vi "RVHR - UI Values.vi"(4 "Default Reporting Settings":T1, 5 "Units":u8, 6 "Initialise?":bool, 7 "Command":enum16{"Set", "Get"}(ring), 8 "error in (no error)":errorcluster, 10 "Reporting IN":T1, 11 "UI Refs":T2) -> (0 "error out":errorcluster, 2 "Reporting Out":T1)   [LabVIEW 2024]
uses:
  Controls/RVHR - Reporting Settings.ctl
  Controls/RVHR - Setting refs.ctl
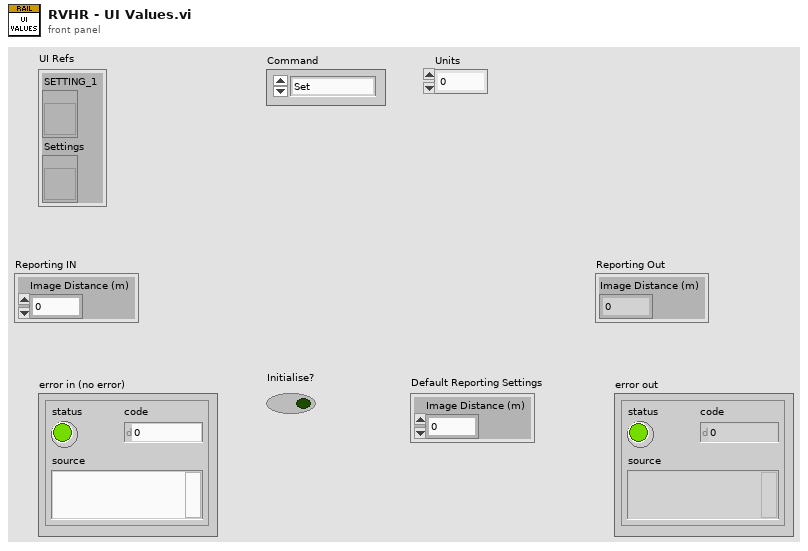
[diagram p1: front panel]
types:
  T1 = typedef "RVHR - Reporting Settings.ctl" = cluster{"Image Distance (m)":dbl}
  T2 = typedef "RVHR - Setting refs.ctl" = cluster{"SETTING_1":refnum<vi>, "Settings":refnum<vi>}
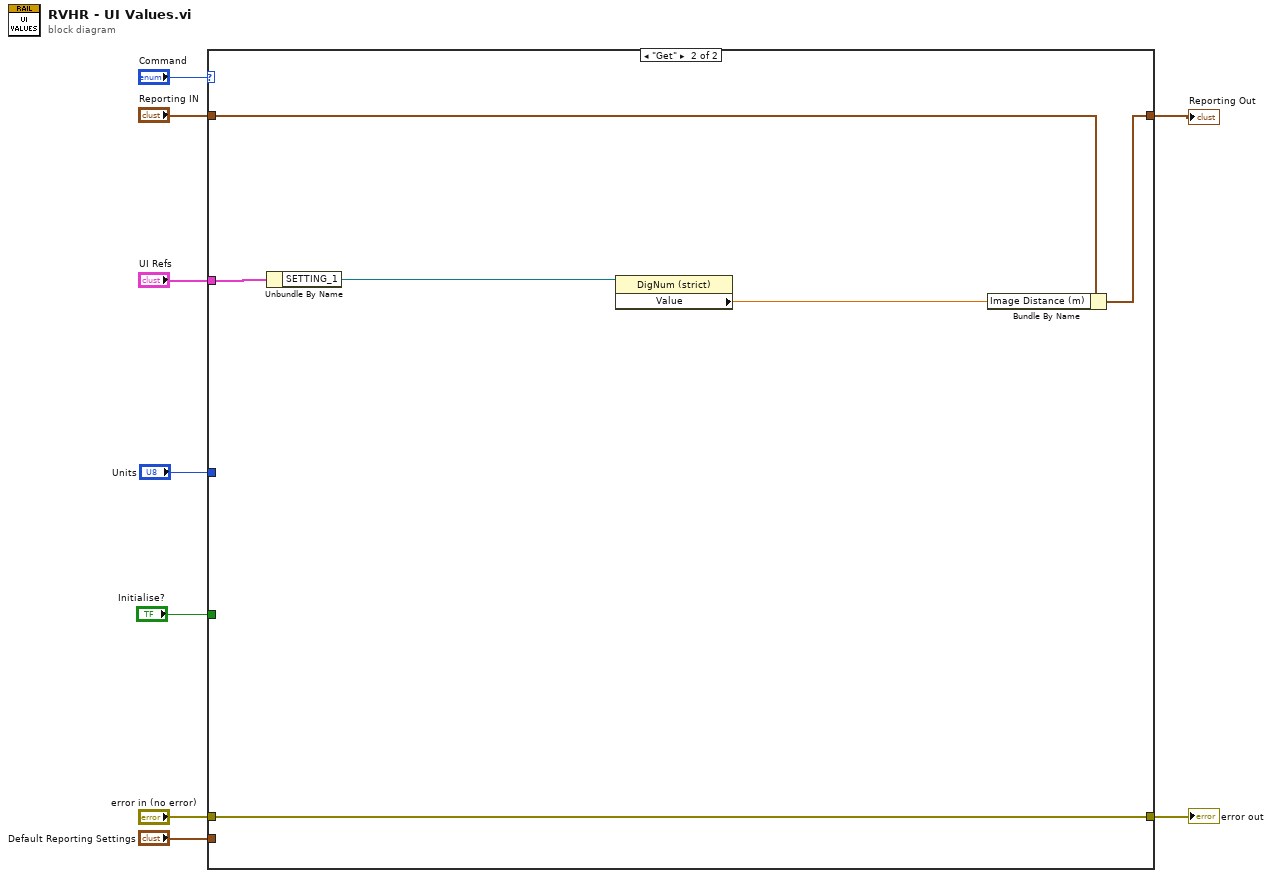
[diagram p0: block diagram]
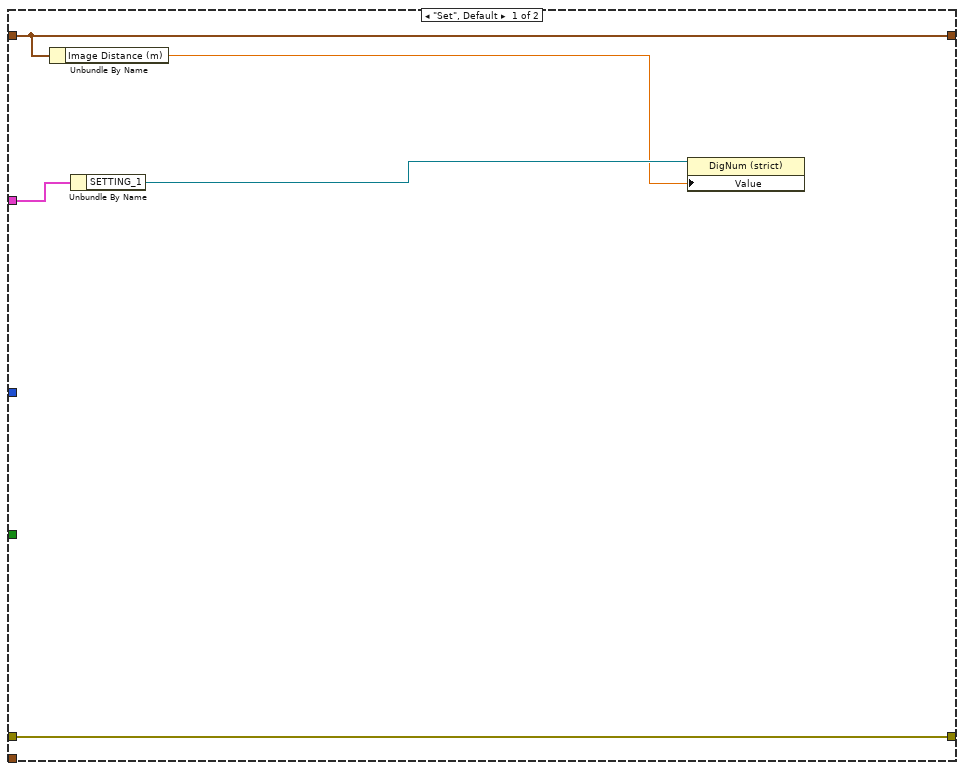
[diagram p2: hidden frame]
diagram:
  n1 = case shown="\"Get\"" "Command" {
    tunnel: "UI Refs" -> [w11 w18]
    tunnel: "Reporting IN" -> [w10 w19]
    tunnel: "error in (no error)" -> [w12 w20]
    tunnel: [w12 w20] -> w8
    tunnel: [w10 w16] -> w9
    tunnel: "Initialise?" -> [_ _]
    tunnel: "Default Reporting Settings" -> [_ _]
    tunnel: "Units" -> [_ _]
    frame "Set", Default {
      n2 = Unbundle By Name(w10) -> ("Image Distance (m)"=w13:dbl)
      n3 = Unbundle By Name(w11) -> ("SETTING_1"=w14:refnum<vi>)
      n4 = property class="DigNum (strict)"(reference=w14, "Value"=w13) -> ()  [unwired: 1 in, 2 out]
    }
    frame "Get" {
      n5 = Unbundle By Name(w18) -> ("SETTING_1"=w17:refnum<vi>)
      n6 = property class="DigNum (strict)"(reference=w17) -> ("Value"=w15:dbl)  [unwired: 1 in, 2 out]
      n7 = Bundle By Name(cluster=w19, "Image Distance (m)"=w15) -> (w16:T1)
    }
  }
  "Reporting Out" <- w9
  "error out" <- w8
